vi "comments-change-eventSD.vi"(1 "cluster in":T1={"Experiments groups"=[], "Kinetics"=[], "Spectrum"=[], "GRAPH EXPERIMENTAL DATA"=[], "kinetics plot names"=[], "spectra plot names"=[], "group"=0, "exp selected"=0, "# exp"=0, "error out"={"status"=FALSE, "code"=0, "source"=""}, "FromToWave"={"FromWave"=0.0, "ToWave"=0.0}, "GRAPH EXPERIMENTAL DATA ref"=refnum, "timedelays"=[0.0, 0.0, 0.0, 0.0, 0.0, 0.0, 0.0, 0.06019061100911815, 0.0521779104562645, 0.045231877429679615, 0.03921051490799832, 0.033990728811568754, 0.029465811603150715, 0.025543260876973825, 0.02214288834180205, 0.01919518054014414, 0.016639877791965713, 0.014424742312398925, 0.012504490320209958, 0.010839866306230088, 0.009396840537117498, 0.008145913389103785, 0.00706151229029317, 0.006121468943269439, 0.005306566140927374, 0.004600144911132549, 0.003987763959109073, 0.0034569044455719407, 0.00299671406541447, 0.0025977851951783253, 0.0022519625739982996, 0.00195217658646366, 0.0016922987392150965, 0.0014670163768006634, 0.0012717240756200802, 0.0011024294957352762, 0.0009556717658856477, 0.0008284507332614981, 0.0007181656316962257, 0.0006225619144775864, 0.0005396851648867825, 0.00046784114226338394, 0.0004055611468220084, 0.0003515719951773376, 0.00030476999279031153, 0.00026419837125694315, 0.00022902772919263772, 0.0001985390768670671, 0.0001721091379728629, 0.00014919760805372974, 0.00012933610911736794], "wavelengths"=[0.0, 0.0, 0.0, 0.0, 0.0, 0.0, 0.0, 0.06019061100911815, 0.0521779104562645, 0.045231877429679615, 0.03921051490799832, 0.033990728811568754, 0.029465811603150715, 0.025543260876973825, 0.02214288834180205, 0.01919518054014414, 0.016639877791965713, 0.014424742312398925, 0.012504490320209958, 0.010839866306230088, 0.009396840537117498, 0.008145913389103785, 0.00706151229029317, 0.006121468943269439, 0.005306566140927374, 0.004600144911132549, 0.003987763959109073, 0.0034569044455719407, 0.00299671406541447, 0.0025977851951783253, 0.0022519625739982996, 0.00195217658646366, 0.0016922987392150965, 0.0014670163768006634, 0.0012717240756200802, 0.0011024294957352762, 0.0009556717658856477, 0.0008284507332614981, 0.0007181656316962257, 0.0006225619144775864, 0.0005396851648867825, 0.00046784114226338394, 0.0004055611468220084, 0.0003515719951773376, 0.00030476999279031153, 0.00026419837125694315, 0.00022902772919263772, 0.0001985390768670671, 0.0001721091379728629, 0.00014919760805372974, 0.00012933610911736794], "Experiment"=refnum, "Commentaires exp"=refnum, "FromToDelay"={"FromDelay"=0.0, "ToDelay"=0.0}}, 2 "NewVal":string) -> (0 "cluster out":T1={"Experiments groups"=[], "Kinetics"=[], "Spectrum"=[], "GRAPH EXPERIMENTAL DATA"=[], "kinetics plot names"=[], "spectra plot names"=[], "group"=0, "exp selected"=0, "# exp"=0, "error out"={"status"=FALSE, "code"=0, "source"=""}, "FromToWave"={"FromWave"=0.0, "ToWave"=0.0}, "GRAPH EXPERIMENTAL DATA ref"=refnum, "timedelays"=[0.0, 0.0, 0.0, 0.0, 0.0, 0.0, 0.0, 0.06019061100911815, 0.0521779104562645, 0.045231877429679615, 0.03921051490799832, 0.033990728811568754, 0.029465811603150715, 0.025543260876973825, 0.02214288834180205, 0.01919518054014414, 0.016639877791965713, 0.014424742312398925, 0.012504490320209958, 0.010839866306230088, 0.009396840537117498, 0.008145913389103785, 0.00706151229029317, 0.006121468943269439, 0.005306566140927374, 0.004600144911132549, 0.003987763959109073, 0.0034569044455719407, 0.00299671406541447, 0.0025977851951783253, 0.0022519625739982996, 0.00195217658646366, 0.0016922987392150965, 0.0014670163768006634, 0.0012717240756200802, 0.0011024294957352762, 0.0009556717658856477, 0.0008284507332614981, 0.0007181656316962257, 0.0006225619144775864, 0.0005396851648867825, 0.00046784114226338394, 0.0004055611468220084, 0.0003515719951773376, 0.00030476999279031153, 0.00026419837125694315, 0.00022902772919263772, 0.0001985390768670671, 0.0001721091379728629, 0.00014919760805372974, 0.00012933610911736794], "wavelengths"=[0.0, 0.0, 0.0, 0.0, 0.0, 0.0, 0.0, 0.06019061100911815, 0.0521779104562645, 0.045231877429679615, 0.03921051490799832, 0.033990728811568754, 0.029465811603150715, 0.025543260876973825, 0.02214288834180205, 0.01919518054014414, 0.016639877791965713, 0.014424742312398925, 0.012504490320209958, 0.010839866306230088, 0.009396840537117498, 0.008145913389103785, 0.00706151229029317, 0.006121468943269439, 0.005306566140927374, 0.004600144911132549, 0.003987763959109073, 0.0034569044455719407, 0.00299671406541447, 0.0025977851951783253, 0.0022519625739982996, 0.00195217658646366, 0.0016922987392150965, 0.0014670163768006634, 0.0012717240756200802, 0.0011024294957352762, 0.0009556717658856477, 0.0008284507332614981, 0.0007181656316962257, 0.0006225619144775864, 0.0005396851648867825, 0.00046784114226338394, 0.0004055611468220084, 0.0003515719951773376, 0.00030476999279031153, 0.00026419837125694315, 0.00022902772919263772, 0.0001985390768670671, 0.0001721091379728629, 0.00014919760805372974, 0.00012933610911736794], "Experiment"=refnum, "Commentaires exp"=refnum, "FromToDelay"={"FromDelay"=0.0, "ToDelay"=0.0}})   [LabVIEW 2015]
uses:
  controls/control-cluster.ctl
  Classes/Experiments_group.lvclass
  Classes/Experiment.lvclass
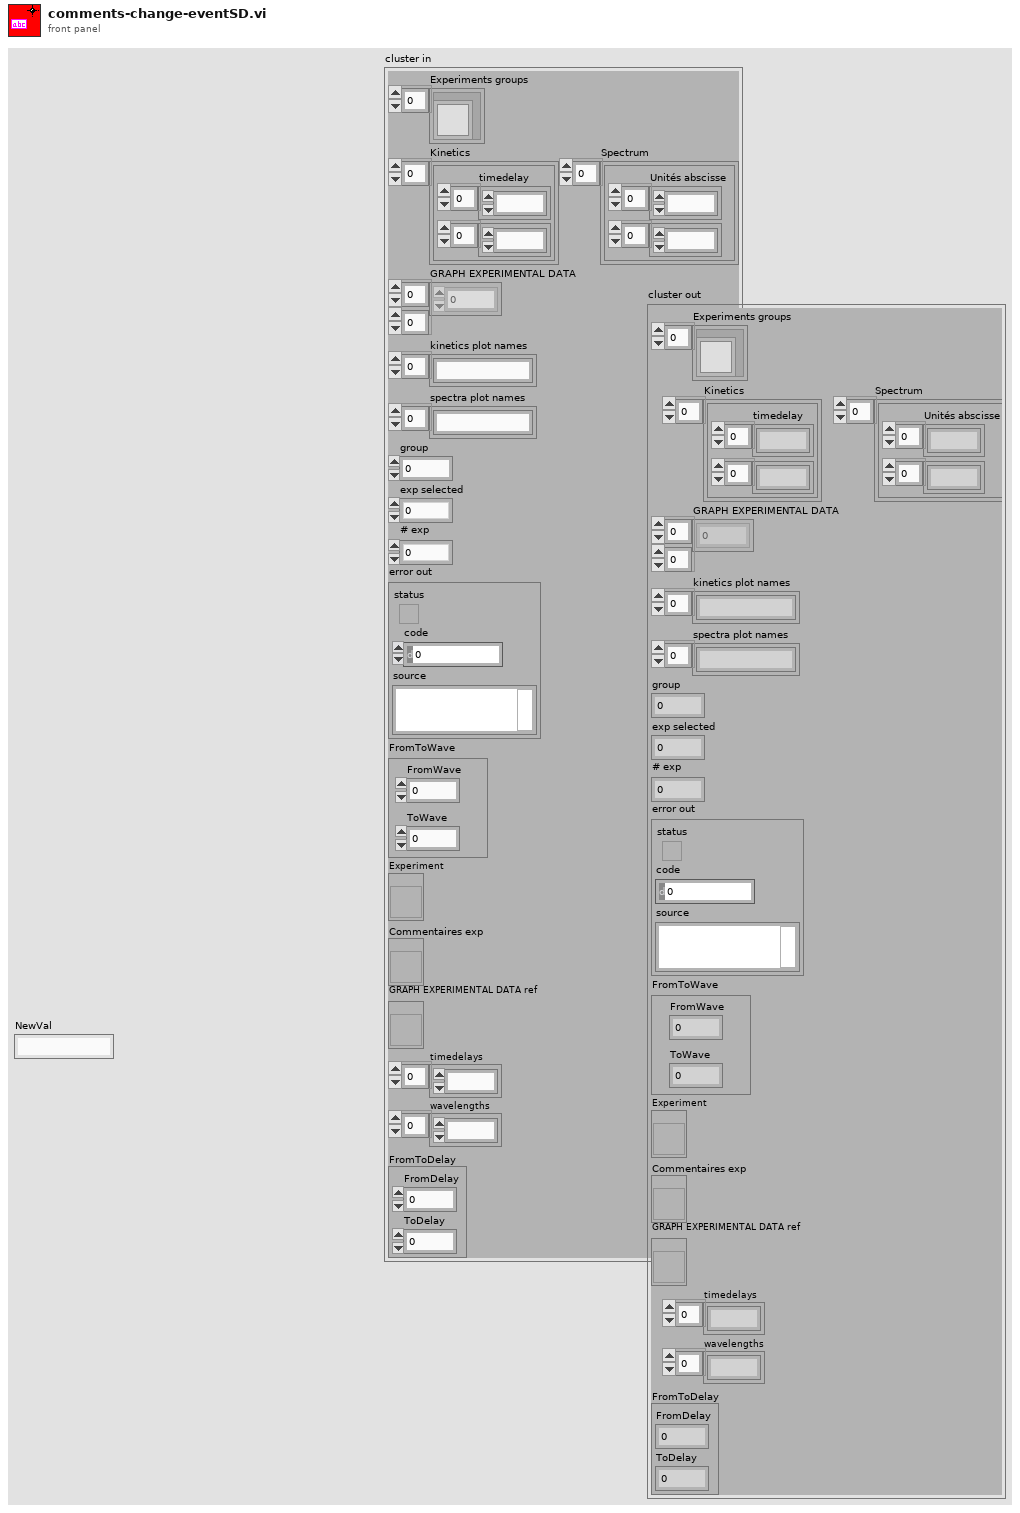
[diagram p1: front panel]
types:
  T1 = typedef "control-cluster.ctl" = cluster{"Experiments groups":refnum<class "Experiments_group.lvclass">[], "Kinetics":cluster{"timedelay":dbl[], dbl[]}[], "Spectrum":cluster{"Unités abscisse":dbl[], dbl[]}[], "GRAPH EXPERIMENTAL DATA":dbl[][], "kinetics plot names":string[], "spectra plot names":string[], "group":i32, "exp selected":i32, "# exp":i32, "error out":errorcluster, "FromToWave":cluster{"FromWave":dbl, "ToWave":dbl}, "GRAPH EXPERIMENTAL DATA ref":refnum<vi>, "timedelays":dbl[], "wavelengths":dbl[], "Experiment":refnum<vi>, "Commentaires exp":refnum<vi>, "FromToDelay":cluster{"FromDelay":dbl, "ToDelay":dbl}}
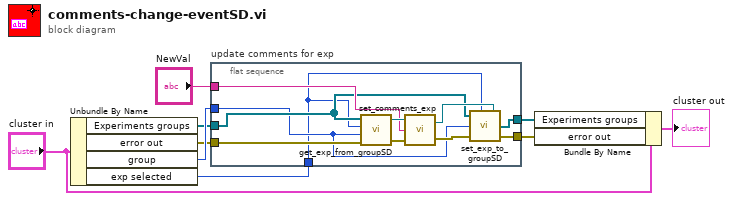
[diagram p0: block diagram]
diagram:
  n1 = Unbundle By Name("cluster in") -> ("Experiments groups"=w4:refnum<class "Experiments_group.lvclass">[], "error out"=w5:errorcluster, "group"=w8:i32, "exp selected"=w9:i32)
  n2 = flat-sequence "update comments for exp" {
    tunnel: "NewVal" -> [w18]
    tunnel: [w12] -> w7
    tunnel: w4 -> [w14]
    tunnel: w5 -> [w20]
    tunnel: [w13] -> w6
    tunnel: w8 -> [w11]
    tunnel: w9 -> [w10]
    frame #0 {
      n3 = call "get_exp_from_groupSD.vi"("error in (no error)"=w20, "group"=w11, "exp selected"=w10, "Experiments groups"=w14) -> ("error out"=w17:errorcluster, "Experiment out"=w19:refnum<class "Experiment.lvclass">)  [unwired: 1 out]
      n4 = call-dynamic "set_comments_exp.vi"("error in (no error)"=w17, "Comments"=w18, "Experiment.lvclass in"=w19) -> ("error out"=w16:errorcluster, "Experiment.lvclass out"=w15:refnum<class "Experiment.lvclass">)
      n5 = call "set_exp_to_groupSD.vi"("Experiments groups"=w14, "exp selected"=w10, "group"=w11, "error in (no error)"=w16, "Experiment in"=w15) -> ("Experiments groups out"=w13:refnum<class "Experiments_group.lvclass">[], "error out"=w12:errorcluster)  [unwired: 1 in]
    }
  }
  n6 = Bundle By Name(cluster="cluster in", "Experiments groups"=w6, "error out"=w7) -> (→"cluster out":T1)
